vi "buffersize_test_optimized.vi"() -> ()   [LabVIEW 2011]
uses:
  <vilib>/Analysis/NI_AALBase.lvlib
panel:
  out "itterations":dbl[](array[numeric])
  out "iterations":i32
  out "curve & length mean":dbl[](array[numeric])
  out "wave read mean":dbl[](array[numeric])
  out "curve & length mean":dbl format="%0.2f"
  out "wave read mean":dbl format="%0.2f"
  out "overall meas time":u32
  in  "averages":i32=10
  out "external iter":i32
  out "internal iter":i32
  out "buffer sizes":i32[](array[numeric])
  out "overall meas times":dbl[](array[numeric])
  in  "buffer size start":i32
  in  "number of diff. buffer sizes":i32
  out "mean overall meas time":dbl format="%0.2f"
  out "Waveform Data":waveform(dbl)(graph)
  in  "VISA resource name":refnum<visa-resource-name>
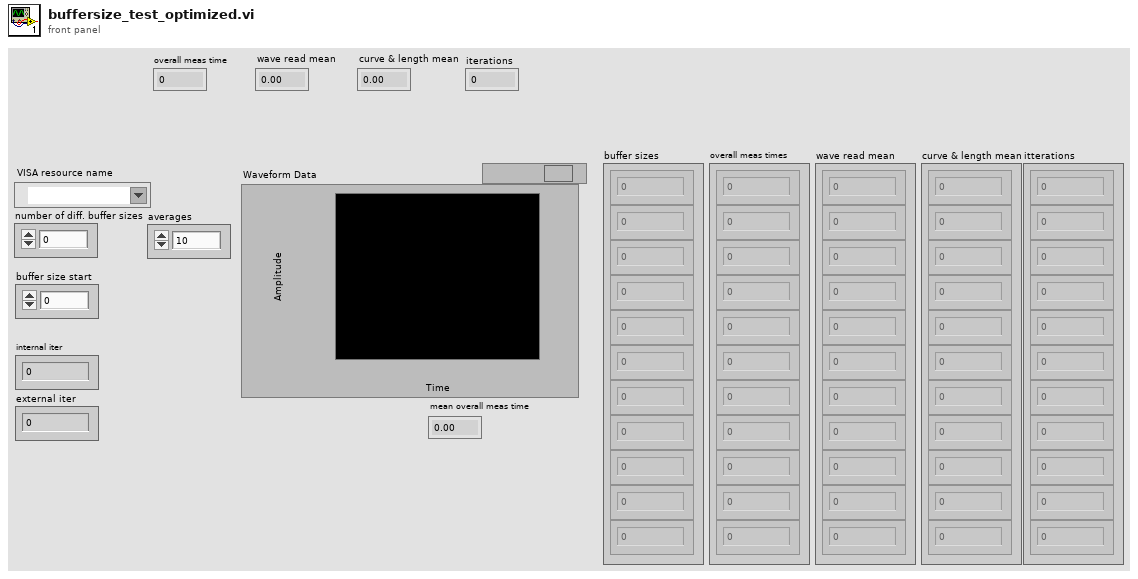
[diagram p1: front panel]
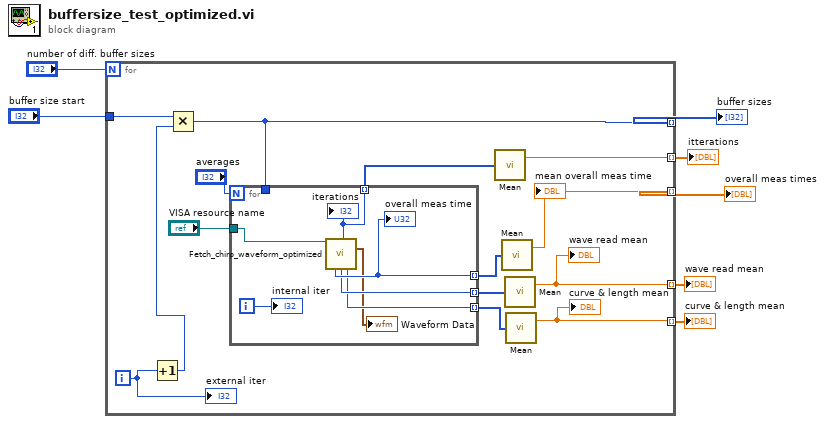
[diagram p0: block diagram]
diagram:
  n1 = for {
    N: "number of diff. buffer sizes" -> [_]
    tunnel: "buffer size start" -> [w19]
    tunnel: [w18] -> w5 mode=indexing
    tunnel: [w17] -> w4 mode=indexing
    tunnel: [w14] -> w3 mode=indexing
    tunnel: [w13] -> w2 mode=indexing
    tunnel: [w8] -> w1 mode=indexing
    i -> [w16]
    n2 = Increment(x=w16) -> (x+1=w15:i32)
    n3 = Multiply(x=w19, y=w15) -> (x*y=w17:i32)
    n4 = for {
      N: "averages" -> [_]
      tunnel: "VISA resource name" -> [w27]
      tunnel: w17 -> [_]
      tunnel: [w26] -> w12 mode=indexing
      tunnel: [w25] -> w11 mode=indexing
      tunnel: [w24] -> w10 mode=indexing
      tunnel: [w22] -> w9 mode=indexing
      i -> [w28]
      n5 = call "Fetch_chirp_waveform_optimized.vi"("VISA resource name"=w27) -> ("iterations"=w22:i32, "Waveform Data"=→"Waveform Data":waveform(dbl), "overall meas time"=w26:u32, "wave meas"=w25:u32, "curvea and length command"=w24:u32)  [unwired: 8 in, 2 out]
      "overall meas time" <- w26
      "iterations" <- w22
      "internal iter" <- w28
    }
    n6 = call <vilib>:"Mean.vi"("X"=w9) -> ("mean"=w8:dbl)  [unwired: 1 out]
    n7 = call <vilib>:"Mean.vi"("X"=w12) -> ("mean"=w18:dbl)  [unwired: 1 out]
    "mean overall meas time" <- w18
    n8 = call <vilib>:"Mean.vi"("X"=w11) -> ("mean"=w14:dbl)  [unwired: 1 out]
    "wave read mean" <- w14
    n9 = call <vilib>:"Mean.vi"("X"=w10) -> ("mean"=w13:dbl)  [unwired: 1 out]
    "curve & length mean" <- w13
    "external iter" <- w16
  }
  "overall meas times" <- w5
  "buffer sizes" <- w4
  "wave read mean" <- w3
  "curve & length mean" <- w2
  "itterations" <- w1
